vi "NovaTech409A_PhaseToCommand.vi"(1 "Novatech Phase [Degrees]":dbl) -> (0 "Novatech Command":u16)   [LabVIEW 2013, in "Novatech 409A.lvlib"]
uses:
  Novatech 409A.lvlib
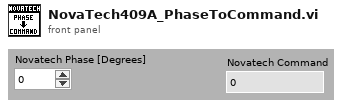
[diagram p1: front panel]
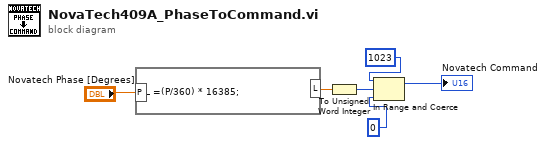
[diagram p0: block diagram]
diagram:
  n1 = formula code="L =(P/360) * 16385;"("P"="Novatech Phase [Degrees]") -> ("L"=w2:dbl)
  n2 = To Unsigned Word Integer(number=w2) -> (unsigned 16bit integer=w3:u16)
  n3 = In Range and Coerce(upper limit=u16 1023, x=w3, lower limit=u16 0) -> (coerced(x)=→"Novatech Command":u16)  [unwired: 1 out]
